vi "line_counter.vi"(2 "iterations until end of fly-back scan segment":u16, 3 "iterations per scan segment":u16, 4 "line counter in":u16, 5 "iteration counter (resonance cycle)":u16) -> (0 "end of line?":bool, 1 "line counter out":u16)   [LabVIEW 2010]
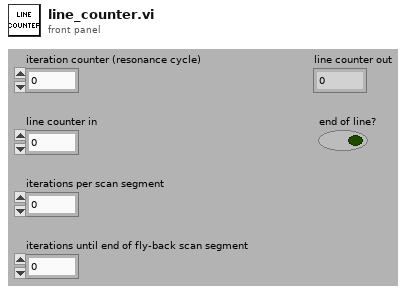
[diagram p1: front panel]
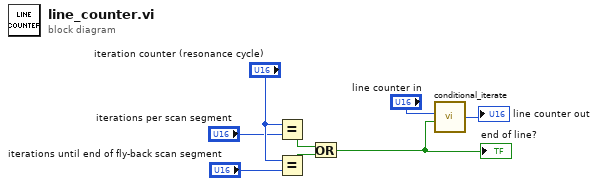
[diagram p0: block diagram]
diagram:
  n1 = Equal?(x="iteration counter (resonance cycle)", y="iterations per scan segment") -> (x = y?=w5:bool)
  n2 = Equal?(x="iteration counter (resonance cycle)", y="iterations until end of fly-back scan segment") -> (x = y?=w4:bool)
  n3 = Or(x=w5, y=w4) -> (x .or. y?=w6:bool)
  "end of line?" <- w6
  n4 = call "conditional_iterate.vi"("iterate?"=w6, "number in"="line counter in") -> ("number out"=→"line counter out":u16)  [unwired: 4 in]
